vi "UltraSound movement.vi"(0 "FPGA VI Reference In":refnum<k20>, 1 "Right Count Length":i16=100, 2 "error in":errorcluster, 3 "DIAG":bool, 4 "STOP?":bool) -> (5 "FPGA VI Reference Out":refnum<k20>, 6 "error out":errorcluster)   [LabVIEW 2014]
uses:
  <vilib>/Utility/error.llb/Error Cluster From Error Code.vi
  <vilib>/rvi/errors/niLvFpgaAdjustHostInterfaceError.vi
  <vilib>/rvi/interface/nirviReadWriteControl/nirviReadWriteControl.xnode
  NiFpgaLv.dll
  <vilib>/rvi/interface/Simulation/niFpgaSimulationCallBeginRW.vi
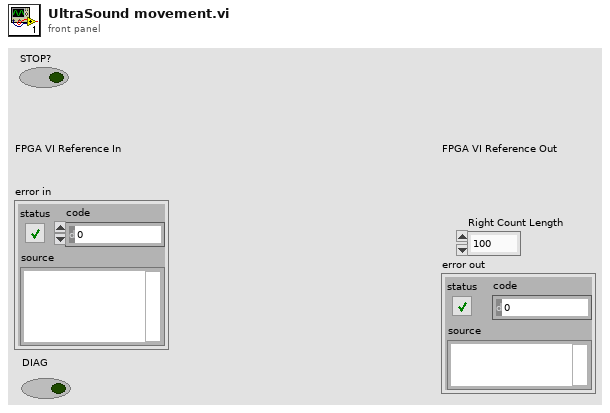
[diagram p1: front panel]
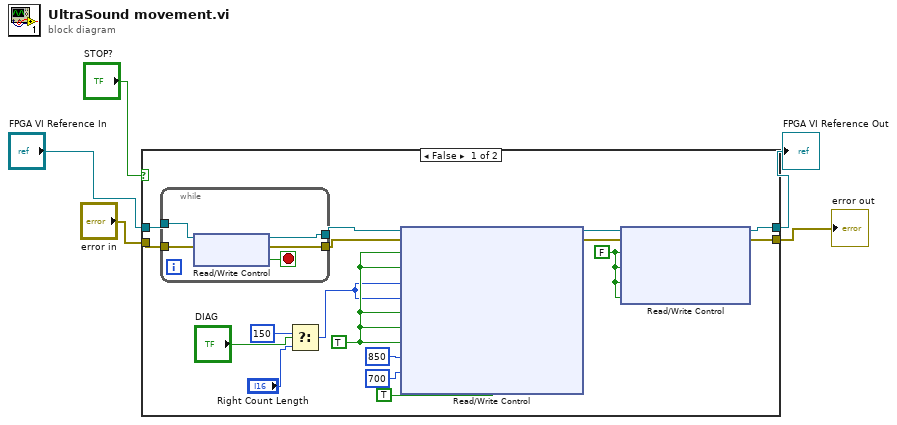
[diagram p0: block diagram]
diagram:
  n1 = case shown="False" "STOP?" {
    tunnel: "FPGA VI Reference In" -> [w9 w29]
    tunnel: "error in" -> [w6 w28]
    tunnel: [w19 w28] -> w3
    tunnel: [w20 w29] -> w2
    frame False {
      w15 = FALSE ("Stop Left")
      w18 = TRUE ("Stop Left")
      n2 = while {
        tunnel: [w26] -> w8
        tunnel: [w25] -> w7
        tunnel: w9 -> [w24]
        tunnel: w6 -> [w23]
        stop <- w27 stop-if-true
        n3 = xnode "Read/Write Control"("FPGA VI Reference In"=w24, "error in"=w23) -> ("FPGA VI Reference Out"=w25:refnum<k20>, "error out"=w26:errorcluster, "Move Stop"=w27:bool)
      }
      n4 = Select(t=i16 150, s="DIAG", f="Right Count Length") -> (s? t:f=w11:i16)
      n5 = xnode "Read/Write Control"("FPGA VI Reference In"=w7, "error in"=w8, "Stop Left"=w18, "Stop Right"=w18, "Left Count Length"=w11, "Right Count Length"=w11, "Left Motor"=w18, "Right Motor"=w18, "reset wheel count (T)"=w18, "Left motor pulse width (uSec)"=850, "Right motor pulse width (uSec)"=700, "Smart Stop"=TRUE) -> ("FPGA VI Reference Out"=w22:refnum<k20>, "error out"=w21:errorcluster)
      n6 = xnode "Read/Write Control"("FPGA VI Reference In"=w22, "error in"=w21, "Stop Left"=w15, "Stop Right"=w15, "reset wheel count (T)"=w15, "Stop motors"=w15) -> ("FPGA VI Reference Out"=w20:refnum<k20>, "error out"=w19:errorcluster)
    }
    frame True {
    }
  }
  "error out" <- w3
  "FPGA VI Reference Out" <- w2
